vi "SubVI_Debug_Arm.vi"(6 "Arm IP Address":string="192.168.10.16", 8 "error in (no error)":errorcluster, 11 "Arm Sampling Rate":u32) -> (0 "error out":errorcluster, 3 "TCP Network Connection out":refnum<k5>)   [LabVIEW 2020]
uses:
  Global 1.vi
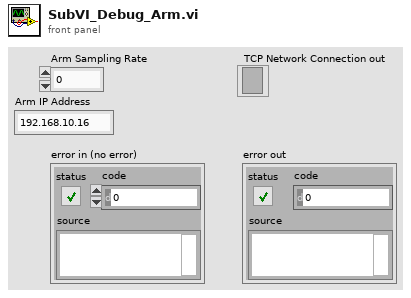
[diagram p1: front panel]
types:
  T1 = enum16{"Standard", "Buffered", "CRLF", "Immediate"}
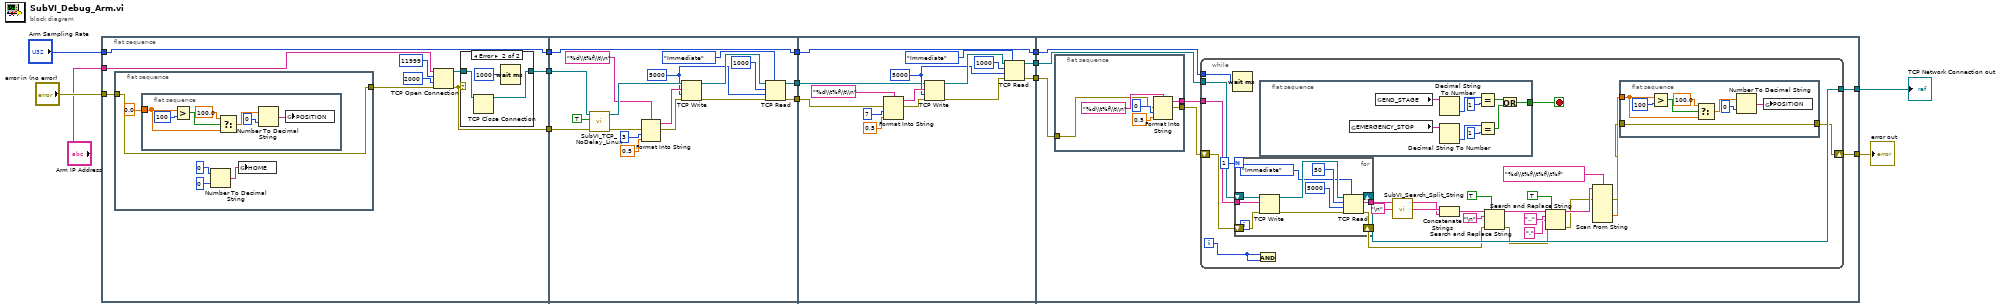
[diagram p0: block diagram]
diagram:
  n1 = flat-sequence {
    tunnel: "error in (no error)" -> [w17]
    tunnel: "Arm Sampling Rate" -> [w16]
    tunnel: [w16] -> w10
    tunnel: [w20] -> w9
    tunnel: [w19] -> w8
    tunnel: "Arm IP Address" -> [w15]
    tunnel: w10 -> [w40]
    tunnel: w9 -> [w56]
    tunnel: w8 -> [w55]
    tunnel: [w40] -> w7
    tunnel: [w45] -> w6
    tunnel: [w44] -> w5
    tunnel: w7 -> [w58]
    tunnel: w6 -> [w62]
    tunnel: w5 -> [w59]
    tunnel: [w58] -> w4
    tunnel: [w61] -> w3
    tunnel: [w60] -> w2
    tunnel: [w78] -> w14
    tunnel: [w77] -> w13
    tunnel: w4 -> [w75]
    tunnel: w3 -> [w74]
    tunnel: w2 -> [w76]
    frame #0 {
      n2 = flat-sequence {
        tunnel: w17 -> [w28]
        tunnel: [w28] -> w18
        frame #0 {
          n3 = flat-sequence {
            tunnel: 0.0 ("Arm_position") -> [w29]
            frame #0 {
              n4 = Greater?(x=w29, y=100) -> (0:w34:bool)
              n5 = Select(t=100.0, s=w34, f=w29) -> (s? t:f=w31:dbl)
              n6 = Number To Decimal String(number=w31, width (-)=i16 0) -> (decimal integer string=w30:string)
              n7 = global write "Global 1.vi" "POSITION"(w30) -> ()
            }
          }
          n8 = Number To Decimal String(number=0, width (-)=i16 0) -> (decimal integer string=w26:string)
          n9 = global write "Global 1.vi" "HOME"(w26) -> ()
        }
      }
      n10 = TCP Open Connection(address=w15, remote port or service name=11999, timeout ms (60000)=2000, error in (no error)=w18) -> (connection ID=w21:refnum<k5>, error out=w20:errorcluster)  [unwired: 1 in]
      n11 = case shown="Error" w20 {
        tunnel: [w36 w37] -> w19
        tunnel: w21 -> [w36 w38]
        frame No Error {
        }
        frame Error {
          n12 = TCP Close Connection(connection ID=w38) -> (connection ID out=w37:refnum<k5>)  [unwired: 2 in, 1 out]
          n13 = Wait (ms)(milliseconds to wait=1000) -> ()  [unwired: 1 out]
        }
      }
    }
    frame #1 {
      w41 = 5000 ("timeout ms (25000)")
      n14 = call "SubVI_TCP_NoDelay_Linux.vi"("error in (no error)"=w56, "TCP_NODELAY (true)"=TRUE, "connID"=w55) -> ("error out"=w49:errorcluster, "connID 2"=w54:refnum<k5>)  [unwired: 3 in]
      n15 = Format Into String(format string="%d\\t%f\\t\\n", error in=w49, 3 ("input 1"), 0.5) -> (resulting string=w50:string, error out=w48:errorcluster)  [unwired: 1 in]
      n16 = TCP Write(connection ID=w54, data in=w50, error in (no error)=w48, 9:w41) -> (connection ID out=w46:refnum<k5>, error out=w47:errorcluster)  [unwired: 1 out]
      n17 = TCP Read(connection ID=w46, bytes to read=1000, error in (no error)=w47, 7:T1."Immediate" ("mode (standard)"), 9:w41) -> (connection ID out=w45:refnum<k5>, error out=w44:errorcluster)  [unwired: 1 out]
    }
    frame #2 {
      w63 = 5000 ("timeout ms (25000)")
      n18 = Format Into String(format string="%d\\t%f\\t\\n", error in=w59, 7 ("input 1"), 0.5) -> (resulting string=w69:string, error out=w68:errorcluster)  [unwired: 1 in]
      n19 = TCP Write(connection ID=w62, data in=w69, error in (no error)=w68, 9:w63) -> (connection ID out=w66:refnum<k5>, error out=w67:errorcluster)  [unwired: 1 out]
      n20 = TCP Read(connection ID=w66, bytes to read=1000, error in (no error)=w67, 7:T1."Immediate" ("mode (standard)"), 9:w63) -> (connection ID out=w60:refnum<k5>, error out=w61:errorcluster)  [unwired: 1 out]
    }
    frame #3 {
      n21 = flat-sequence {
        tunnel: [w140] -> w79
        tunnel: w74 -> [w136]
        tunnel: [w135] -> w73
        frame #0 {
          n22 = Format Into String(format string="%d\\t%f\\t\\n", error in=w136, 0 ("input 1"), 0.5) -> (resulting string=w140:string, error out=w135:errorcluster)  [unwired: 1 in]
        }
      }
      n23 = while {
        shift-right: [w82] -> w78
        shift-left: w73 -> [w105]
        tunnel: w79 -> [w104]
        tunnel: [w106] -> w77
        tunnel: w76 -> [w90]
        tunnel: w75 -> [w88]
        i -> [w81]
        stop <- w87 stop-if-true
        n24 = Wait (ms)(milliseconds to wait=w88) -> ()  [unwired: 1 out]
        n25 = for {
          N: 1 -> [_]
          tunnel: w104 -> [w113]
          tunnel: [w109] -> w97
          shift-right: [w107] -> w86
          shift-left: w105 -> [w116]
          shift-right: [w117] -> w106
          shift-left: w90 -> [w108]
          n26 = TCP Write(connection ID=w108, data in=w113, error in (no error)=w116) -> (connection ID out=w115:refnum<k5>, error out=w114:errorcluster)  [unwired: 1 in, 1 out]
          n27 = TCP Read(connection ID=w115, bytes to read=50, error in (no error)=w114, 7:T1."Immediate" ("mode (standard)"), 9:5000 ("timeout ms (25000)")) -> (connection ID out=w117:refnum<k5>, data out=w109:string, error out=w107:errorcluster)
        }
        n28 = And(x=w81, y=w81) -> ()  [unwired: 1 out]
        n29 = flat-sequence {
          tunnel: [w126] -> w87
          frame #0 {
            n30 = global read "Global 1.vi" "EMERGENCY_STOP"() -> (w129:string)
            n31 = global read "Global 1.vi" "END_STAGE"() -> (w134:string)
            n32 = Decimal String To Number(string=w134) -> (number=w133:i32)  [unwired: 2 in, 1 out]
            n33 = Decimal String To Number(string=w129) -> (number=w131:i32)  [unwired: 2 in, 1 out]
            n34 = Equal?(x=w133, y=1) -> (x = y?=w127:bool)
            n35 = Equal?(x=w131, y=1) -> (x = y?=w128:bool)
            n36 = Or(x=w127, y=w128) -> (x .or. y?=w126:bool)
          }
        }
        n37 = call <userlib>:"SubVI_Search_Split_String.vi"("search string/char (-)"="\n", "string"=w97) -> ("substring after match"=w102:string, "substring before match"=w101:string)  [unwired: 1 in, 1 out]
        n38 = Concatenate Strings(w102, w101) -> (w103:string)
        n39 = Search and Replace String(replace all?=TRUE ("replace all? (F)"), input string=w103, search string="\n", error in=w86) -> (result string=w95:string, error out=w85:errorcluster)  [unwired: 4 in, 2 out]
        n40 = Search and Replace String(replace all?=TRUE ("replace all? (F)"), input string=w95, search string="..", replace string="." ("replace string (\"\")"), error in=w85) -> (result string=w93:string, error out=w84:errorcluster)  [unwired: 3 in, 2 out]
        n41 = Scan From String(format string="%d\\t%f\\t%f\\t%f", input string=w93, error in=w84) -> (error out=w83:errorcluster, output 3=w89:dbl)  [unwired: 8 in, 2 out]
        n42 = flat-sequence {
          tunnel: w89 -> [w119]
          tunnel: w83 -> [w118]
          tunnel: [w118] -> w82
          frame #0 {
            n43 = Greater?(x=w119, y=100) -> (0:w124:bool)
            n44 = Select(t=100.0, s=w124, f=w119) -> (s? t:f=w121:dbl)
            n45 = Number To Decimal String(number=w121, width (-)=i16 0) -> (decimal integer string=w120:string)
            n46 = global write "Global 1.vi" "POSITION"(w120) -> ()
          }
        }
      }
    }
  }
  "error out" <- w14
  "TCP Network Connection out" <- w13
